vi "CANOpen Enter Node ID.vi"(8 "error in (no error)":errorcluster, 11 "Node Ptr":u64 format="%.0x") -> (0 "error out":errorcluster, 1 "Cancelled?":bool, 2 "Node ID Out":string, 3 "Item Ref out":T1 format="%.0x", 5 "Node ID out":u8=1 min=1 max=127 step=1)   [LabVIEW 2021, in "CANOpen Addon System Explorer.lvlib"]
uses:
  CANOpen Addon System Explorer.lvlib
  <vilib>/NI VeriStand/Custom Device API/Custom Device Item Ref.ctl
  <vilib>/NI VeriStand/Custom Device API/Custom Device API.lvlib
panel:
  in  "Cancel Button":bool
  in  "OK Button":bool
  in  "Node ID":u8=1 min=1 max=127 step=1
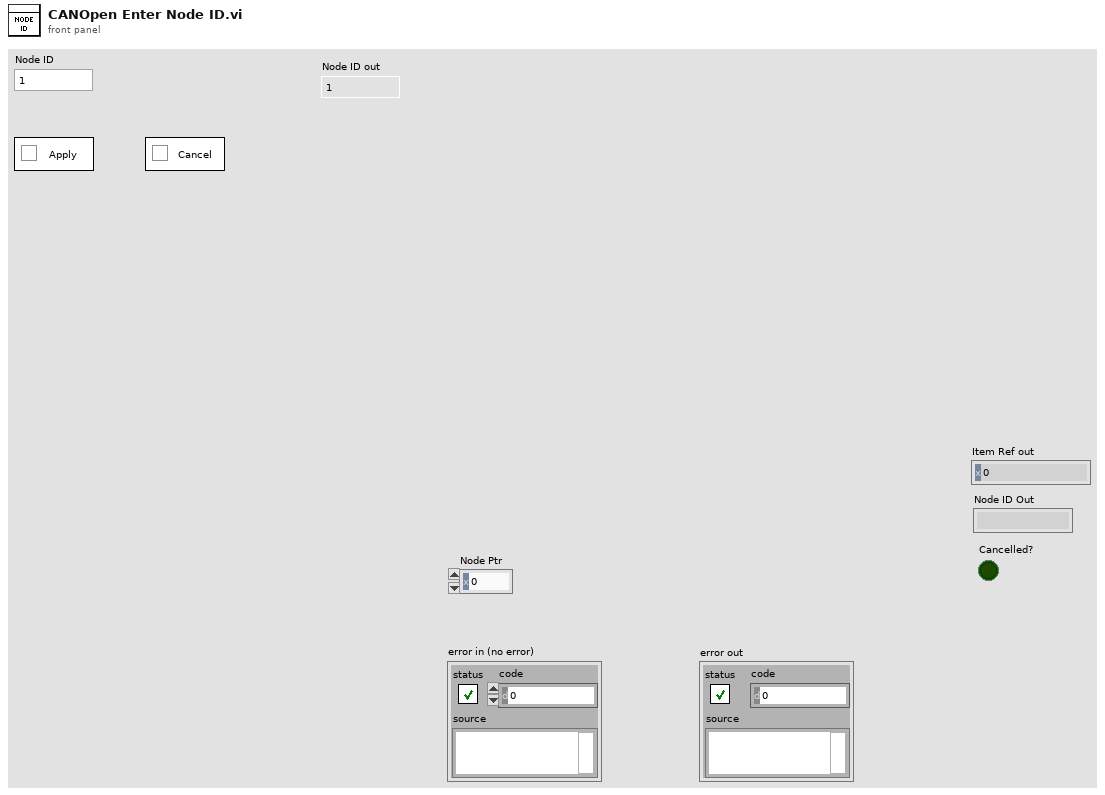
[diagram p1: front panel]
types:
  T1 = typedef "Custom Device API.lvlib/Custom Device Item Ref.ctl" = u64
  T2 = typedef "Custom Device API.lvlib/Custom Device Item Info.ctl" = cluster{"Name":string, "Is Channel":bool, "GUID":string, "Is Waveform":bool}
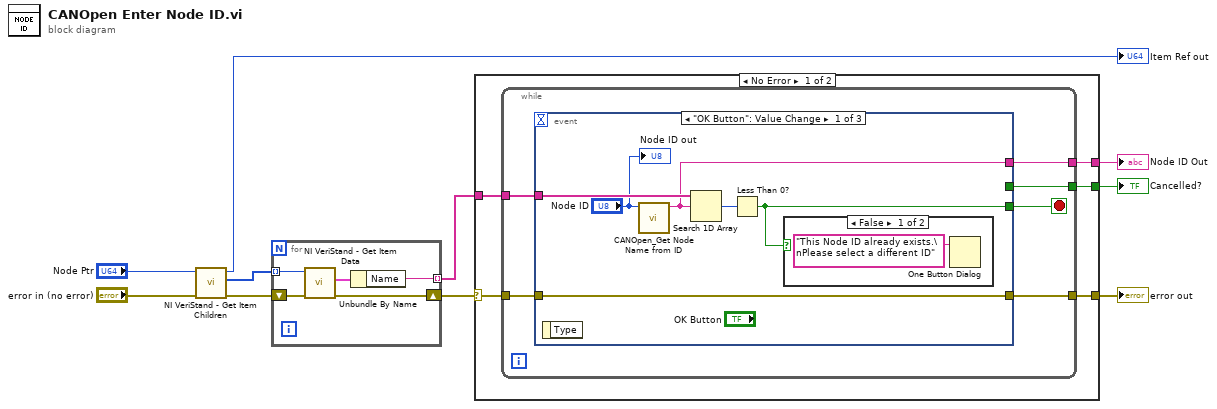
[diagram p0: block diagram]
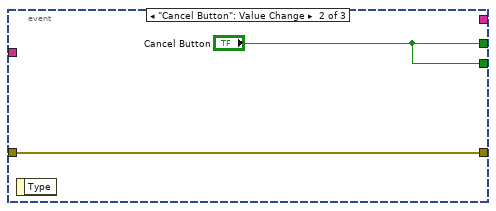
[diagram p3: hidden frame]
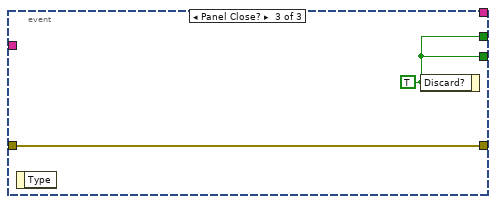
[diagram p4: hidden frame]
diagram:
  n1 = call <vilib>:"NI VeriStand - Get Item Children.vi"("error in (no error)"="error in (no error)", "Item Ref in"="Node Ptr") -> ("error out"=w7:errorcluster, "Child Refs"=w5:T1[], "Item Ref out"=→"Item Ref out":T1)  [unwired: 6 in, 1 out]
  n2 = for {
    tunnel: w5 -> [w14] mode=indexing
    tunnel: [w11] -> w4 mode=indexing
    shift-right: [w12] -> w6
    shift-left: w7 -> [w13]
    n3 = call <vilib>:"NI VeriStand - Get Item Data.vi"("error in (no error)"=w13, "Item Ref in"=w14) -> ("error out"=w12:errorcluster, "Item Info"=w15:T2)  [unwired: 6 in, 2 out]
    n4 = Unbundle By Name(w15) -> ("Name"=w11:string)
  }
  n5 = case shown="No Error" w6 {
    selector: w6 -> [w16 w38]
    tunnel: [w20 w38] -> w10
    tunnel: w4 -> [w19 _]
    tunnel: [w18 _] -> w9
    tunnel: [w17 _] -> w8
    frame No Error {
      n6 = while {
        tunnel: [w26] -> w20
        tunnel: w16 -> [w25]
        tunnel: w19 -> [w24]
        tunnel: [w22] -> w18
        tunnel: [w21] -> w17
        stop <- w23 stop-if-true
        n7 = event shown="[0] \"OK Button\": Value Change" {
          selector: _ -> [_ _ _]
          dyn-events: _ -> [_ _ _]
          timeout: _ -> [_ _ _]
          tunnel: [w27 w35 w37] -> w26
          tunnel: w25 -> [w27 w35 w37]
          tunnel: w24 -> [w32 _ _]
          tunnel: [w31 "Cancel Button" w36] -> w23
          tunnel: [w28 _ _] -> w22
          tunnel: [_ "Cancel Button" w36] -> w21
          event "OK Button": Value Change {
            n8 = event-data() -> ()  [unwired: 1 in, 1 out]
            n9 = call "CANOpen_Get Node Name from ID.vi"("Node ID"="Node ID") -> ("Node ID Name"=w28:string)  [unwired: 10 in]
            n10 = Search 1D Array(1D array=w32, element=w28) -> (index of element=w30:i32)  [unwired: 1 in]
            n11 = Less Than 0?(x=w30) -> (x < 0?=w31:bool)
            n12 = case shown="False" w31 {
              frame False {
                n13 = One Button Dialog(message="This Node ID already exists.\nPlease select a different ID") -> ()  [unwired: 1 in, 1 out]
              }
              frame True {
              }
            }
            "Node ID out" <- "Node ID"
          }
          event "Cancel Button": Value Change {
            n14 = event-data() -> ()  [unwired: 1 in, 1 out]
          }
          event Panel Close? {
            w36 = TRUE ("Discard?")
            n15 = event-data() -> ()  [unwired: 1 in, 1 out]
            n16 = event-data("Discard?"=w36) -> ()  [unwired: 1 in, 1 out]
          }
        }
      }
    }
    frame Error {
    }
  }
  "error out" <- w10
  "Cancelled?" <- w8
  "Node ID Out" <- w9
